vi "Create All Message Queues.vi"(8 "error in (no error)":errorcluster) -> (0 "error out":errorcluster, 3 "Message Queues out":T1)   [LabVIEW 2013, in "synergia Message Queue.lvlib"]
doc: "This VI creates and initializes all the message queues for your application. If your application requires more than one message queue, right-click the \"Message Queues\" constant above and select Open Type Def. Add the new Message Queue(s) to the type definition, then initialize them in this VI."
uses:
  synergia Message Queue.lvlib
  All Message Queues.ctl
  Message Cluster.ctl
  Enqueue Message (Single).vi
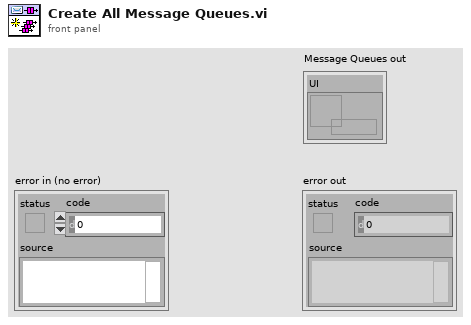
[diagram p1: front panel]
types:
  T1 = typedef "synergia Message Queue.lvlib/All Message Queues.ctl" = cluster{"UI":refnum<queue>}
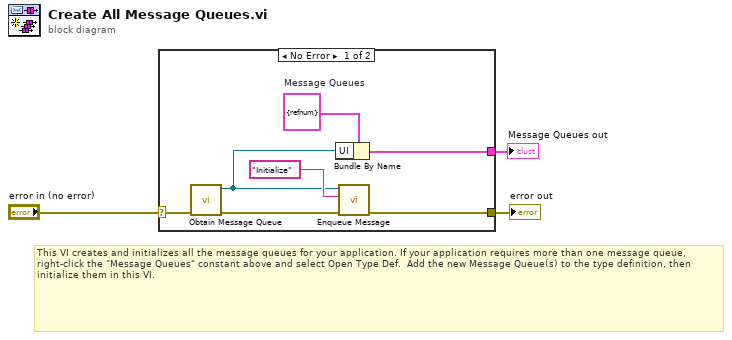
[diagram p0: block diagram]
diagram:
  # "This VI creates and initializes all the message queues for your application. If your application requires more than one message queue, right-click the \"Message Queues\" constant above and select Open Type Def.  Add the new Message Queue(s) to the type definition, then initialize them in this VI."
  n1 = case shown="No Error" "error in (no error)" {
    selector: "error in (no error)" -> [w7 w11]
    tunnel: [w10 w11] -> w3
    tunnel: [w8 _] -> w2
    frame No Error {
      w9 = T1 {"UI"=refnum}  # Message Queues
      n2 = call "Obtain Message Queue.vi"("error in (no error)"=w7) -> ("error out"=w6:errorcluster, "Message Queue"=w4:refnum<queue>)  [unwired: 9 in]
      n3 = Bundle By Name(cluster=w9, "UI"=w4) -> (w8:T1)
      n4 = call-poly "Enqueue Message.vi"("error in (no error)"=w6, "Message"="Initialize", "Message Queue"=w4) -> ("error out"=w10:errorcluster)  [unwired: 7 in, 1 out]
    }
    frame Error {
    }
  }
  "Message Queues out" <- w2
  "error out" <- w3
